vi "tsdb_get_can_db_info.vi"(6 "path in":path, 7 "QueryType":T1 items=["DT_STR_Network_Name", "DT_STR_DBC_FileName", "DT_INT_Protocol_Type", "DT_INT_3", "DT_INT_4", "DT_INT_5", "DT_INT_6", "DT_INT_7", "DT_INT_8", "DT_INT_9", "DT_INT_Signal_List_Count", "DT_INT_CAN_Message_List_Count", "DT_INT_CANFD_Message_List_Count", "DT_INT_CANJ1939_Message_List_Count", "DT_INT_Node_List_Count", "DT_INT_EnvVar_List_Count", "DT_INT_ValTab_List_Count", "DT_INT_17", "DT_INT_18", "DT_INT_19", "DT_INT_Signal_List_Message_ID", "DT_INT_Signal_List_Value_Type", "DT_INT_Signal_List_Is_Motorola", "DT_INT_Signal_List_ValTab_Index", "DT_INT_Signal_List_Mux_Type", "DT_INT_Signal_List_Mux_Value", "DT_INT_Signal_List_Layout_Start", "DT_INT_Signal_List_Length", "DT_DBL_Signal_List_Factor", "DT_DBL_Signal_List_Offset", "DT_DBL_Signal_List_InitValue", "DT_DBL_Signal_List_Min", "DT_DBL_Signal_List_Max", "DT_STR_Signal_List_Name", "DT_STR_Signal_List_Unit", "DT_STR_Signal_List_Comment", "DT_INT_Signal_List_Message_Index", "DT_INT_Signal_List_Message_Type", "DT_STR_Signal_List_Struct", "DT_INT_39", "DT_INT_CAN_Message_List_Type", "DT_INT_CAN_Message_List_DLC", "DT_INT_CAN_Message_List_ID", "DT_INT_CAN_Message_List_CycleTime", "DT_STR_CAN_Message_List_Name", "DT_STR_CAN_Message_List_Comment", "DT_INT_CAN_Message_List_TX_Node_Index", "DT_INT_CAN_Message_List_Owned_Signal_List_Count", "DT_INT_CAN_Message_List_Owned_Signal_List_Signal_Index", "DT_STR_CAN_Message_List_Struct", "DT_INT_50", "DT_INT_51", "DT_INT_52", "DT_INT_53", "DT_INT_54", "DT_INT_55", "DT_INT_56", "DT_INT_57", "DT_INT_58", "DT_INT_59", "DT_INT_CANFD_Message_List_Type", "DT_INT_CANFD_Message_List_DLC", "DT_INT_CANFD_Message_List_ID", "DT_INT_CANFD_Message_List_CycleTime", "DT_STR_CANFD_Message_List_Name", "DT_STR_CANFD_Message_List_Comment", "DT_INT_CANFD_Message_List_TX_Node_Index", "DT_INT_CANFD_Message_List_Owned_Signal_List_Count", "DT_INT_CANFD_Message_List_Owned_Signal_List_Signal_Index", "DT_INT_CANFD_Message_List_BRS", "DT_STR_CANFD_Message_List_Struct", "DT_INT_71", "DT_INT_72", "DT_INT_73", "DT_INT_74", "DT_INT_75", "DT_INT_76", "DT_INT_77", "DT_INT_78", "DT_INT_79", "DT_INT_J1939_Message_List_Type", "DT_INT_J1939_Message_List_DLC", "DT_INT_J1939_Message_List_ID", "DT_INT_J1939_Message_List_CycleTime", "DT_STR_J1939_Message_List_Name", "DT_STR_J1939_Message_List_Comment", "DT_INT_J1939_Message_List_TX_Node_Index", "DT_INT_J1939_Message_List_Owned_Signal_List_Count", "DT_INT_J1939_Message_List_Owned_Signal_List_Signal_Index", "DT_STR_J1939_Message_List_Struct", "DT_INT_90", "DT_INT_91", "DT_INT_92", "DT_INT_93", "DT_INT_94", "DT_INT_95", "DT_INT_96", "DT_INT_97", "DT_INT_98", "DT_INT_99", "DT_INT_Node_List_Address", "DT_STR_Node_List_Name", "DT_STR_Node_List_Comment", "DT_INT_Node_List_TX_CAN_Message_List_Count", "DT_INT_Node_List_TX_CAN_Message_List_Message_Index", "DT_INT_Node_List_RX_CAN_Message_List_Count", "DT_INT_Node_List_RX_CAN_Message_List_Message_Index", "DT_INT_Node_List_TX_FD_Message_List_Count", "DT_INT_Node_List_TX_FD_Message_List_Message_Index", "DT_INT_Node_List_RX_FD_Message_List_Count", "DT_INT_Node_List_RX_FD_Message_List_Message_Index", "DT_INT_Node_List_TX_J1939_Message_List_Count", "DT_INT_Node_List_TX_J1939_Message_List_Message_Index", "DT_INT_Node_List_RX_J1939_Message_List_Count", "DT_INT_Node_List_RX_J1939_Message_List_Message_Index", "DT_INT_Node_List_TX_Signal_List_Count", "DT_INT_Node_List_TX_Signal_List_Signal_Index", "DT_INT_Node_List_RX_Signal_List_Count", "DT_INT_Node_List_RX_Signal_List_Signal_Index", "DT_STR_Node_List_Struct", "DT_INT_120", "DT_INT_121", "DT_INT_122", "DT_INT_123", "DT_INT_124", "DT_INT_125", "DT_INT_126", "DT_INT_127", "DT_INT_128", "DT_INT_129", "DT_INT_EnvVar_List_Value_Type", "DT_DBL_EnvVar_List_MIN", "DT_DBL_EnvVar_List_MAX", "DT_DBL_EnvVar_List_Init_Value", "DT_STR_EnvVar_List_Name", "DT_STR_EnvVar_List_Unit", "DT_STR_EnvVar_List_Comment", "DT_STR_EnvVar_List_Struct", "DT_INT_138", "DT_INT_139", "DT_INT_ValTab_List_Item_List_Count", "DT_INT_ValTab_List_Item_List_Name", "DT_DBL_ValTab_List_Item_List_Value", "DT_STR_ValTab_List_Struct"], 8 "error in":errorcluster, 9 "ASubIndex":i32, 10 "AIndex":i32, 11 "ADatabaseId":u32) -> (0 "error out":errorcluster, 1 "ANumValue":i32, 2 "AValue":string, 3 "AId":u32, 4 "path out":path)   [LabVIEW 2014]
uses:
  <vilib>/Utility/importsl/GetValueByPointer/GetValueByPointer.xnode
  <vilib>/Utility/importsl/GetValueByPointer/datatype.ctl
  Typedef/QueryType.ctl
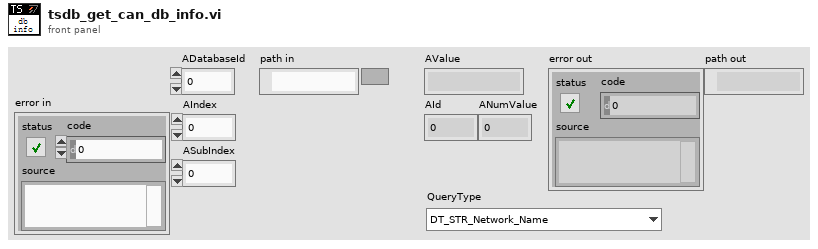
[diagram p1: front panel]
types:
  T1 = typedef "QueryType.ctl" = i32
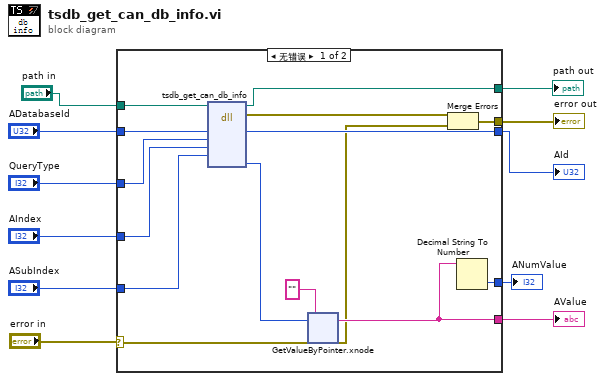
[diagram p0: block diagram]
diagram:
  n1 = case shown="无错误" "error in" {
    selector: "error in" -> [w20 w41]
    tunnel: "ADatabaseId" -> [w26 w40]
    tunnel: "QueryType" -> [w25 _]
    tunnel: "AIndex" -> [w24 _]
    tunnel: "ASubIndex" -> [w23 _]
    tunnel: [w16 _] -> w7
    tunnel: [w18 w41] -> w5
    tunnel: [w17 w40] -> w4
    tunnel: [w15 _] -> w3
    tunnel: "path in" -> [w13 w39]
    tunnel: [w12 w39] -> w1
    frame No Error {
      n2 = dll-call lib="D:/Program Files (x86)/TOSUN/TSMaster/bin/TSMaster.dll" fn="tsdb_get_can_db_info"(path in=w13, "ADatabaseId"=w26, "AType"=w25, "AIndex"=w24, "ASubIndex"=w23) -> (path out=w12:path, error out=w19:errorcluster, "ADatabaseId"=w17:u32, "AValueAddr"=w22:u64)  [unwired: 7 in]
      n3 = xnode "GetValueByPointer.xnode"("Pointer"=w22, "InputType"="", "ErrorIn"=w20) -> ("Output"=w16:string, "ErrorOut"=w14:errorcluster)  [unwired: 1 in]
      n4 = Merge Errors(w19, w14) -> (w18:errorcluster)
      n5 = Decimal String To Number(string=w16) -> (number=w15:i32)  [unwired: 2 in, 1 out]
    }
    frame Error {
    }
  }
  "error out" <- w5
  "AValue" <- w7
  "AId" <- w4
  "ANumValue" <- w3
  "path out" <- w1
